vi "get_version_path.vi"(8 "error in (no error)":errorcluster, 10 "project_file":path, 11 "custom_path":path) -> (0 "error out":errorcluster, 3 "lv_build_version_path":path)   [LabVIEW 2015, in "lv-builder-default.lvlib"]
uses:
  lv-builder-default.lvlib
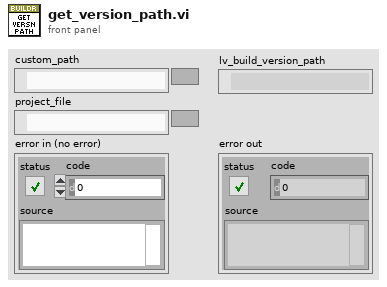
[diagram p1: front panel]
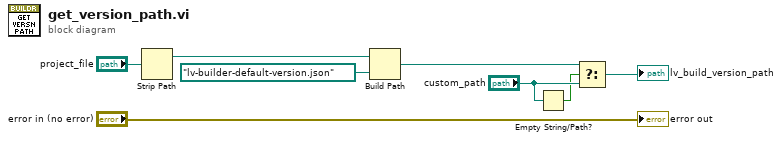
[diagram p0: block diagram]
diagram:
  n1 = Strip Path(path="project_file") -> (stripped path=w1:path)  [unwired: 1 out]
  n2 = Build Path(base path=w1, name or relative path=path "lv-builder-default-version.json" ("system directory")) -> (appended path=w6:path)
  n3 = Empty String/Path?(string/path="custom_path") -> (empty?=w3:bool)
  n4 = Select(t=w6, s=w3, f="custom_path") -> (s? t:f=→"lv_build_version_path":path)
  "error out" <- "error in (no error)"
